vi "MovingAverage.vi"(10 "Datapoint":dbl, 11 "Moving Average Length":i32=1 min=1) -> (3 "Moving Average":dbl)   [LabVIEW 2014]
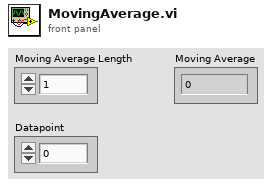
[diagram p1: front panel]
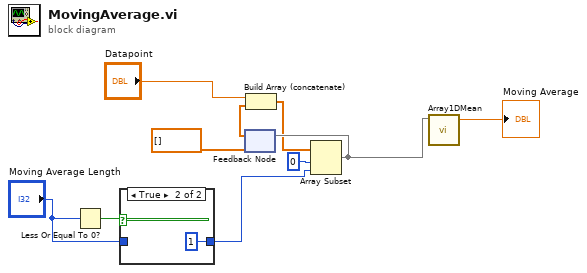
[diagram p0: block diagram]
diagram:
  n1 = Less Or Equal To 0?(x="Moving Average Length") -> (x <= 0?=w3:bool)
  n2 = case shown="True" w3 {
    tunnel: [w11 1 ("Moving Average Length")] -> w1
    tunnel: "Moving Average Length" -> [w11 _]
    frame False {
    }
    frame True {
    }
  }
  n3 = feedback #1(dbl[] []) -> (w6:dbl[])
  n4 = Build Array (concatenate)("Datapoint", w6) -> (w4:dbl[])
  n5 = Array Subset(array=w4, index=0, length=w1) -> (w9:dbl[])
  n6 = feedback-in #1(w9) -> ()
  n7 = call "Array1DMean.vi"("Array"=w9) -> ("Numeric Control"=→"Moving Average":dbl)  [unwired: 10 in]
